vi "Permutate Array.vi"(11 "unsigned byte array in":u8[](array[numeric])) -> (3 "unsigned byte array out":u8[][](array[numeric]))   [LabVIEW 2020]
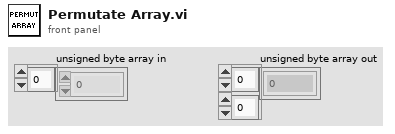
[diagram p1: front panel]
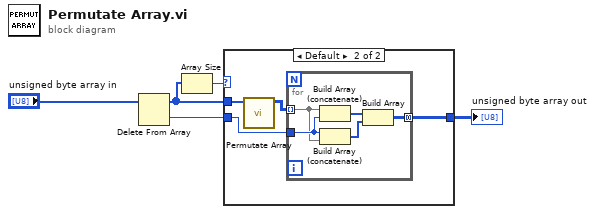
[diagram p0: block diagram]
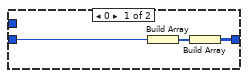
[diagram p2: hidden frame]
diagram:
  n1 = Delete From Array(array="unsigned byte array in") -> (deleted portion=w4:u8, array with subset deleted=w2:u8[])  [unwired: 2 in]
  n2 = Array Size(array=w2) -> (size(s)=w1:i32)
  n3 = case shown="Default" w1 {
    tunnel: w4 -> [w8 w9]
    tunnel: [w6 w10] -> w3
    tunnel: w2 -> [_ w12]
    frame 0 {
      n4 = Build Array(w8) -> (w7:u8[])
      n5 = Build Array(w7) -> (w6:u8[][])
    }
    frame Default {
      n6 = call "Permutate Array.vi"("unsigned byte array in"=w12) -> ("unsigned byte array out"=w11:u8[][])  [unwired: 10 in]
      n7 = for {
        tunnel: w11 -> [w14] mode=indexing
        tunnel: [w16] -> w10 mode=concatenating
        tunnel: w9 -> [w15]
        n8 = Build Array (concatenate)(w14, w15) -> (w17:u8[])
        n9 = Build Array (concatenate)(w15, w14) -> (w13:u8[])
        n10 = Build Array(w17, w13) -> (w16:u8[][])
      }
    }
  }
  "unsigned byte array out" <- w3
